vi "PH_Connection.connect to PSDB.vi"(2 "error in":errorcluster, 3 "PSDB Credentials":cluster{"PW":string, "ID":string, "DS":string}={"PW"="N/A", "ID"="N/A", "DS"="N/A"}) -> (0 "error out":errorcluster, 1 "connection reference":T1)   [LabVIEW 2014, in "PH_Common.lvlib"]
doc: "This VI opens a connection to the PHELIX shot data base."
uses:
  PH_Common.lvlib
  <vilib>/addons/database/Connection.llb/Conn ObjectReference.ctl
  <vilib>/addons/database/NI_Database_API.lvlib
  User/Eisenbarth/psdb_lv/PSDB.lvlib
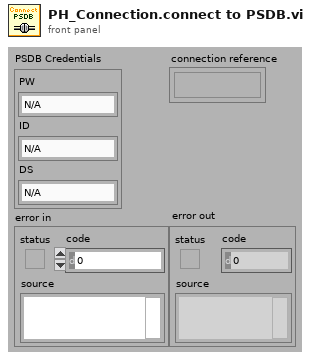
[diagram p1: front panel]
types:
  T1 = typedef "NI_Database_API.lvlib/Conn ObjectReference.ctl" = refnum<k1>
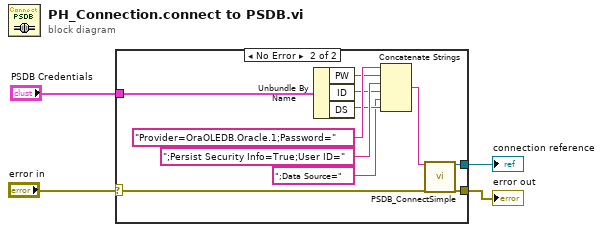
[diagram p0: block diagram]
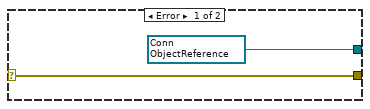
[diagram p2: hidden frame]
diagram:
  n1 = case shown="No Error" "error in" {
    selector: "error in" -> [w6 w16]
    tunnel: [w5 w17] -> w2
    tunnel: [w6 w15] -> w3
    tunnel: "PSDB Credentials" -> [_ w11]
    frame Error {
      w5 = T1 refnum items=["Connection"] ("connection reference")
    }
    frame No Error {
      n2 = Unbundle By Name(w11) -> ("PW"=w10:string, "ID"=w8:string, "DS"=w9:string)
      n3 = Concatenate Strings("Provider=OraOLEDB.Oracle.1;Password=", w10, ";Persist Security Info=True;User ID=" ("string"), w8, ";Data Source=" ("string"), w9) -> (w12:string)
      n4 = call "PSDB_ConnectSimple.vi"("Connection Information"=w12, "error in (no error)"=w16) -> ("connection reference"=w17:T1, "error out"=w15:errorcluster)  [unwired: 16 in]
    }
  }
  "error out" <- w3
  "connection reference" <- w2
